vi "Parse Registers into IPs.vi"(6 "IP Types":refnum<class "Engine Simulation IP.lvclass">[](array[class]), 7 "engine simulation session in":refnum<class "Engine Simulation Session.lvclass">, 8 "error in (no error)":errorcluster, 9 "Version":T1, 11 "Registers LUT":variant) -> (0 "error out":errorcluster, 3 "IPs":refnum<class "Engine Simulation IP.lvclass">[](array[class]))   [LabVIEW 2013, in "Engine Simulation Session.lvclass"]
uses:
  Engine Simulation Session.lvclass
  Engine Simulation IP.lvclass
  Bitfile Major Version.ctl
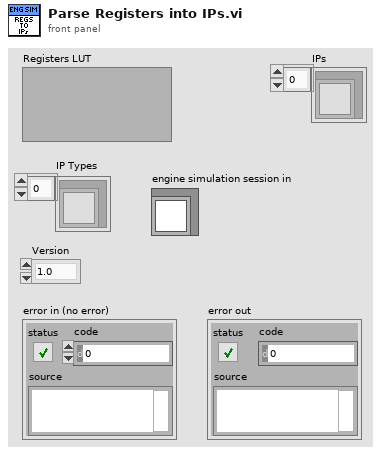
[diagram p1: front panel]
types:
  T1 = typedef "Engine Simulation Session.lvclass/Bitfile Major Version.ctl" = enum16{"1.0", "1.1", "1.2", "1.3"}
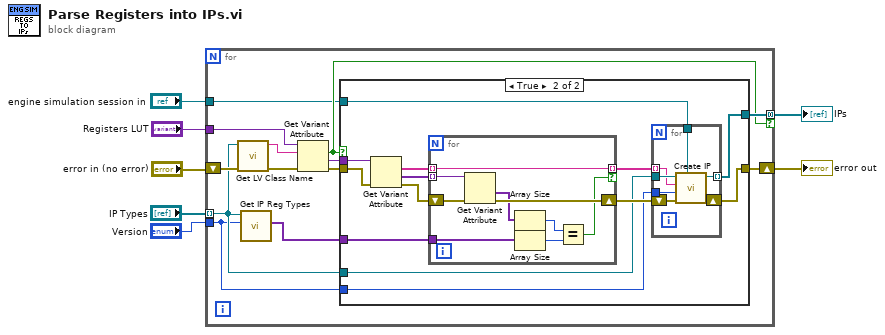
[diagram p0: block diagram]
diagram:
  n1 = for {
    tunnel: [w20] -> w7 mode=concatenating if=w10
    tunnel: "Registers LUT" -> [w19]
    tunnel: "IP Types" -> [w11] mode=indexing
    shift-right: [w17] -> w5
    shift-left: "error in (no error)" -> [w18]
    tunnel: "Version" -> [w9]
    tunnel: "engine simulation session in" -> [w8]
    n2 = call <vilib>:"Get LV Class Name.vi"("error in (no error)"=w18, "object"=w11) -> ("error out"=w14:errorcluster, "class name"=w13:string)  [unwired: 8 in]
    n3 = call-dynamic "Get IP Reg Types.vi"("Version"=w9, "Engine Simulation IP in"=w11) -> ("IP Regs"=w12:variant[])  [unwired: 8 in, 1 out]
    n4 = Get Variant Attribute(Variant=w19, name=w13, error in=w14) -> (found=w10:bool, value=w15:variant, error out=w16:errorcluster)  [unwired: 1 in, 1 out]
    n5 = case shown="True" w10 {
      tunnel: w16 -> [w21 w33]
      tunnel: w15 -> [_ w34]
      tunnel: [w21 w27] -> w17
      tunnel: w12 -> [_ w32]
      tunnel: w11 -> [_ w26]
      tunnel: w9 -> [_ w25]
      tunnel: [_ w24] -> w20
      tunnel: w8 -> [_ w22]
      frame False {
      }
      frame True {
        n6 = Get Variant Attribute(Variant=w34, error in=w33) -> (names=w30:string[], values=w29:variant[], error out=w31:errorcluster)  [unwired: 2 in, 1 out]
        n7 = for {
          tunnel: w32 -> [w50]
          shift-right: [w46] -> w28
          shift-left: w31 -> [w47]
          tunnel: w30 -> [w44] mode=indexing
          tunnel: w29 -> [w48] mode=indexing
          tunnel: [w44] -> w23 mode=indexing if=w43
          n8 = Get Variant Attribute(Variant=w48, error in=w47) -> (values=w45:variant[], error out=w46:errorcluster)  [unwired: 2 in, 2 out]
          n9 = Array Size(array=w45) -> (size(s)=w49:i32)
          n10 = Array Size(array=w50) -> (size(s)=w42:i32)
          n11 = Equal?(x=w49, y=w42) -> (x = y?=w43:bool)
        }
        n12 = for {
          shift-right: [w37] -> w27
          shift-left: w28 -> [w41]
          tunnel: w23 -> [w39] mode=indexing
          tunnel: w26 -> [w40]
          tunnel: w25 -> [w38]
          tunnel: [w36] -> w24 mode=indexing
          tunnel: w22 -> [w35]
          n13 = call-dynamic "Create IP.vi"("session"=w35, "error in (no error)"=w41, "EST version enum"=w38, "Name"=w39, "Engine Simulation IP in"=w40) -> ("error out"=w37:errorcluster, "Engine Simulation IP out"=w36:refnum<class "Engine Simulation IP.lvclass">)  [unwired: 5 in]
        }
      }
    }
  }
  "IPs" <- w7
  "error out" <- w5
